vi "spectro.vi"() -> ()   [LabVIEW 2016]
uses:
  <vilib>/Analysis/baseanly.llb/Mean (DBL).vi
  <vilib>/Utility/file.llb/Write Delimited Spreadsheet (string).vi
  <vilib>/Utility/file.llb/Write Delimited Spreadsheet (DBL).vi
  <vilib>/Analysis/NI_AALBase.lvlib
panel:
  in  "stop":bool
  in  "Tab Control":enum32{"medir", "Mover"}(tab)
  out "Offset":dbl
  out "val act":dbl
  out "Valor y prom":dbl
  in  "num. med.":dbl
  out "XY Graph":cluster{dbl[], dbl[]}(graph)
  in  "iniciar":bool
  out "posicion":dbl
  in  "intervalo":dbl
  in  "Fin":dbl=100.0 min=100.0 max=15000.0
  in  "Inicio":dbl
  in  "offset":dbl=2000.0
  out "Longitud de onda actual":dbl
  in  "Mover":bool
  in  "Mover Monocromador":dbl
  in  "aceptar posición act.":bool
  in  "Posición actual":dbl
  # "Mover Monocromador"
  # "Definir Posición Actual"
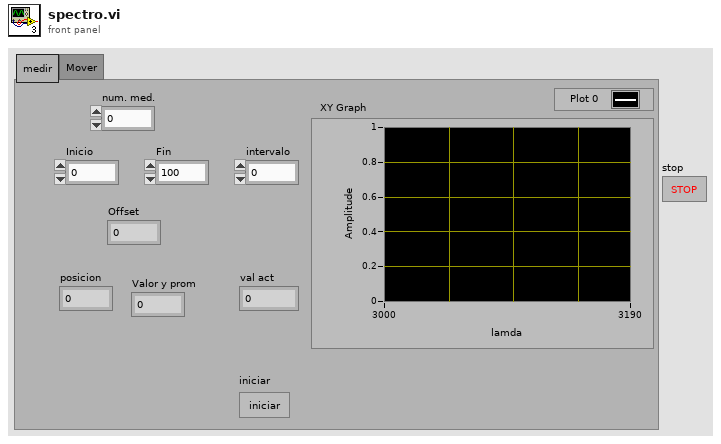
[diagram p1: front panel]
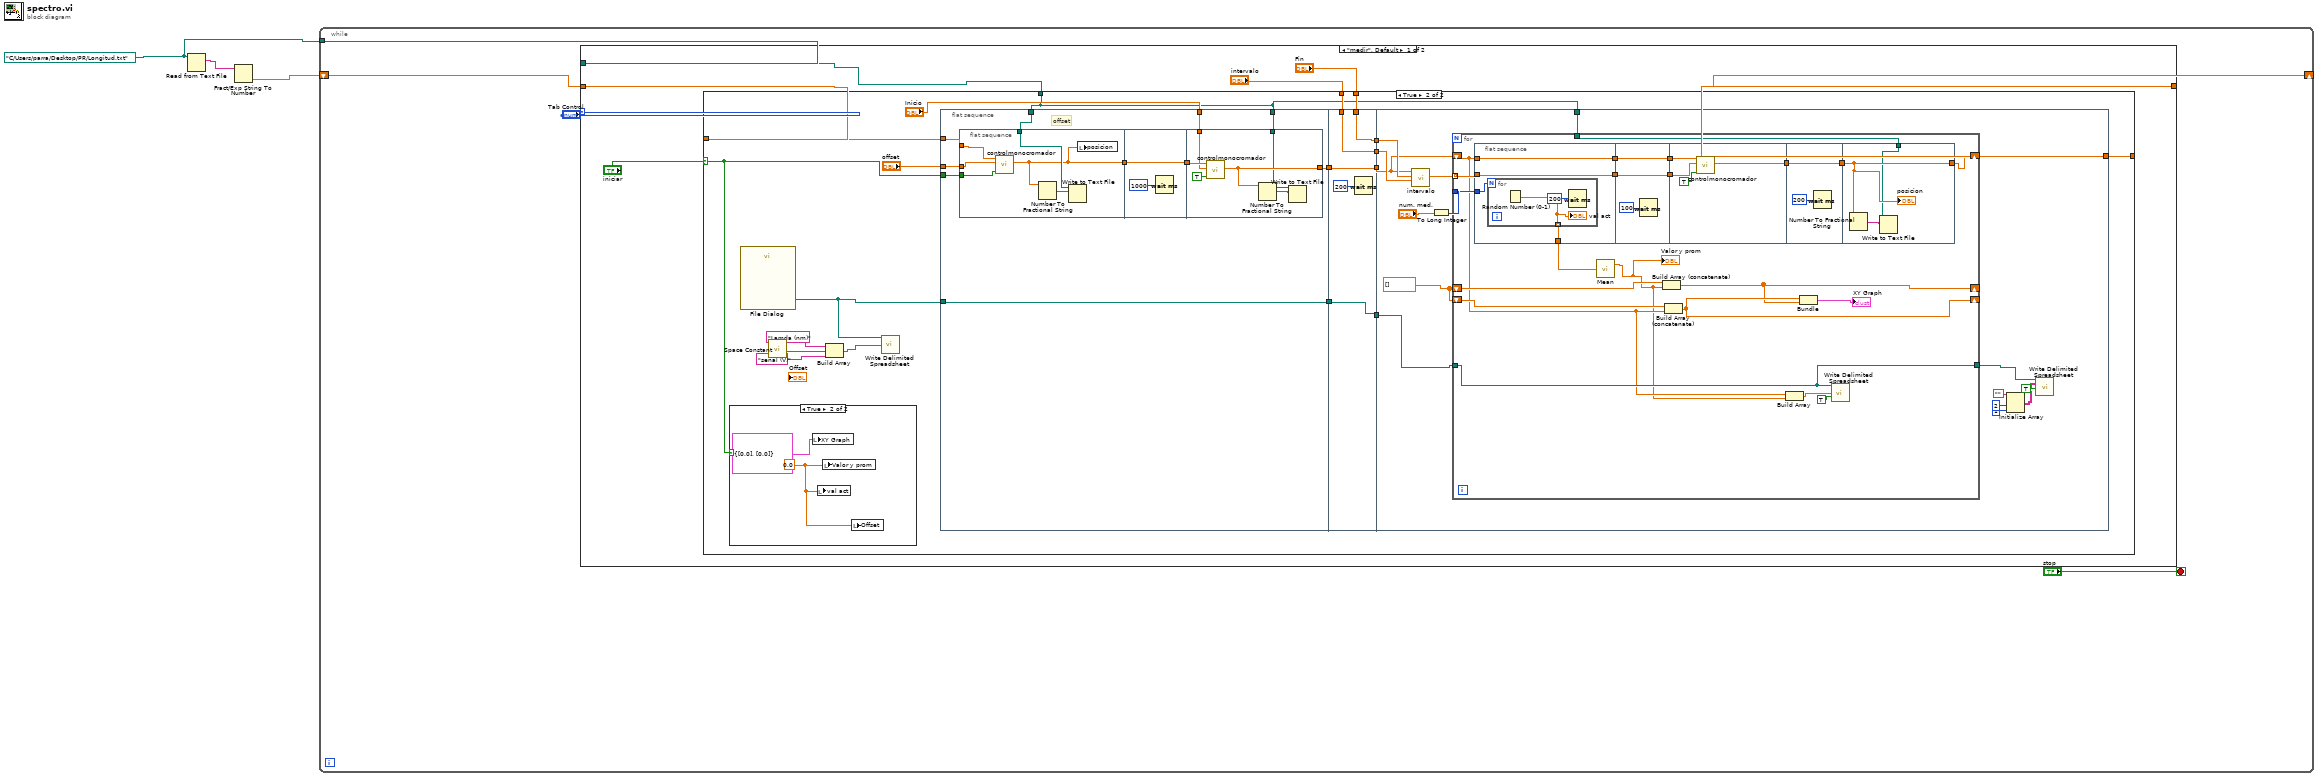
[diagram p0: block diagram]
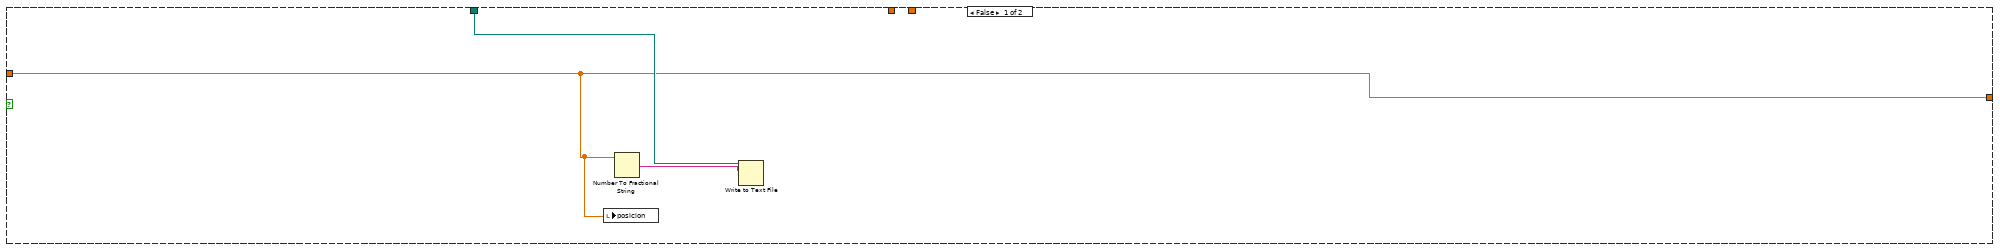
[diagram p2: hidden frame]
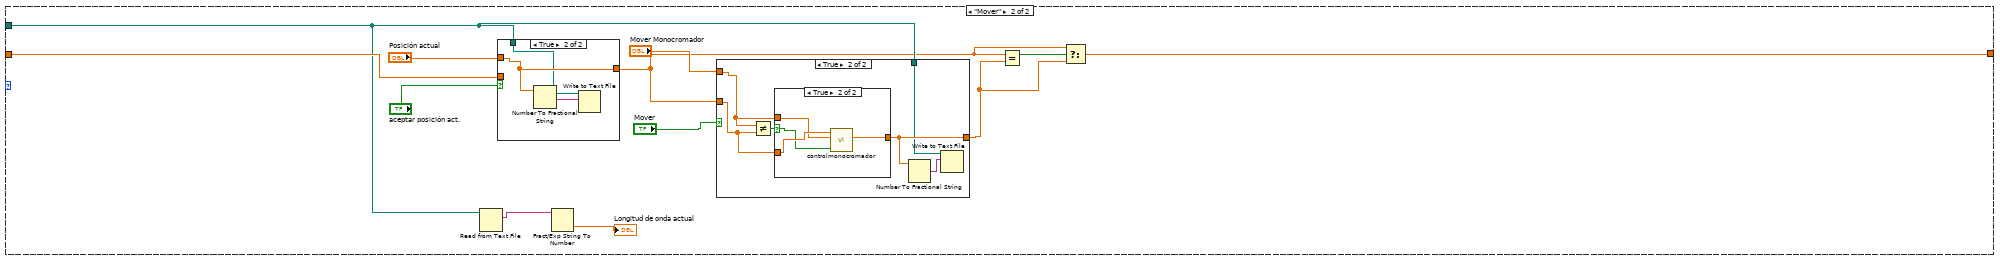
[diagram p4: hidden frame]
diagram:
  w1 = path "C:/Users/parra/Desktop/PR/Longitud.txt" ("file (use dialog)")
  n1 = Read from Text File(file (use dialog)=w1) -> (text=w3:string)  [unwired: 3 in, 3 out]
  n2 = Fract/Exp String To Number(string=w3) -> (number=w2:dbl)  [unwired: 3 in, 1 out]
  n3 = while {
    shift-right: [w4] -> _
    shift-left: w2 -> [w5]
    tunnel: w1 -> [w6]
    stop <- "stop" stop-if-true
    n4 = case shown="\"medir\", Default" "Tab Control" {
      tunnel: w6 -> [w13 w127]
      tunnel: w5 -> [w14 w132]
      tunnel: [w10 w123] -> w4
      frame "medir", Default {
        n5 = case shown="True" "iniciar" {
          selector: "iniciar" -> [_ w19]
          tunnel: w14 -> [w15 w35]
          tunnel: w13 -> [w17 w27]
          tunnel: "Fin" -> [_ w30]
          tunnel: "intervalo" -> [_ w28]
          tunnel: [w15 w26] -> w10
          frame False {
            n6 = local write "posicion"(w15) -> ()
            n7 = Number To Fractional String(number=w15) -> (F-format string=w16:string)  [unwired: 3 in]
            n8 = Write to Text File(file (use dialog)=w17, text=w16) -> ()  [unwired: 2 in, 3 out]
          }
          frame True {
            n9 = case shown="True" w19 {
              frame False {
              }
              frame True {
                w37 = 0.0 ("Valor y prom")
                n10 = local write "XY Graph"(cluster{dbl[], dbl[]} {[0.0], [0.0]} ("XY Graph")) -> ()
                n11 = local write "val act"(w37) -> ()
                n12 = local write "Valor y prom"(w37) -> ()
                n13 = local write "Offset"(w37) -> ()
              }
            }
            n14 = call "File Dialog"() -> ("selected path"=w23:path)  [unwired: 12 in, 3 out]
            n15 = call <vilib>:"Space Constant.vi"() -> ("String"=w21:string)
            n16 = Build Array("Lamda (nm)", w21, "señal (V)" ("element")) -> (w18:string[])
            n17 = call-poly <vilib>:"Write Delimited Spreadsheet.vi"("file path (dialog if empty)"=w23, "1D data"=w18) -> ()  [unwired: 12 in, 2 out]
            n18 = flat-sequence {
              tunnel: w35 -> [w48]
              tunnel: "offset" -> [w47]
              tunnel: w19 -> [w46]
              tunnel: w27 -> [w45]
              tunnel: "Inicio" -> [w42]
              tunnel: w27 -> [w41]
              tunnel: [w40] -> w33
              tunnel: w23 -> [w39]
              tunnel: [w39] -> w24
              tunnel: w33 -> [w67]
              tunnel: [w67] -> w32
              tunnel: [w65] -> w31
              tunnel: w30 -> [w65]
              tunnel: w28 -> [w64]
              tunnel: [w64] -> w29
              tunnel: [w63] -> w25
              tunnel: w24 -> [w63]
              tunnel: w32 -> [w80]
              tunnel: w31 -> [w83]
              tunnel: w29 -> [w82]
              tunnel: w27 -> [w79]
              tunnel: [w78] -> w26
              tunnel: w25 -> [w74]
              frame #0 {
                # "offset"
                n19 = flat-sequence {
                  tunnel: w48 -> [w54]
                  tunnel: w47 -> [w53]
                  tunnel: w46 -> [w49]
                  tunnel: w45 -> [w51]
                  tunnel: [w50] -> w44
                  tunnel: w44 -> [w56]
                  tunnel: [w56] -> w43
                  tunnel: w43 -> [w62]
                  tunnel: w42 -> [w61]
                  tunnel: [w59] -> w40
                  tunnel: w41 -> [w58]
                  frame #0 {
                    n20 = call "controlmonocromador.vi"(8:"inicio"=w49, "fin"=w53, 11:"inicio"=w54) -> ("Longitud actual"=w50:dbl)  [unwired: 8 in]
                    n21 = Number To Fractional String(number=w50) -> (F-format string=w52:string)  [unwired: 3 in]
                    n22 = Write to Text File(file (use dialog)=w51, text=w52) -> ()  [unwired: 2 in, 3 out]
                    n23 = local write "posicion"(w50) -> ()
                  }
                  frame #1 {
                    n24 = Wait (ms)(milliseconds to wait=u32 1000) -> ()  [unwired: 1 out]
                  }
                  frame #2 {
                    n25 = call "controlmonocromador.vi"(8:"inicio"=TRUE ("inicio"), "fin"=w61, 11:"inicio"=w62) -> ("Longitud actual"=w59:dbl)  [unwired: 8 in]
                    n26 = Number To Fractional String(number=w59) -> (F-format string=w60:string)  [unwired: 3 in]
                    n27 = Write to Text File(file (use dialog)=w58, text=w60) -> ()  [unwired: 2 in, 3 out]
                  }
                }
              }
              frame #1 {
                n28 = Wait (ms)(milliseconds to wait=u32 200) -> ()  [unwired: 1 out]
              }
              frame #2 {
                w75 = dbl[] []
                n29 = call "intervalo.vi"("Intervalo"=w82, "Final"=w83, "inicio"=w80) -> ("Array"=w81:dbl[])  [unwired: 8 in]
                n30 = To Long Integer(number="num. med.") -> (32bit integer=w76:i32)
                n31 = for {
                  tunnel: w81 -> [w104] mode=indexing
                  shift-right: [w91] -> w78
                  shift-left: w80 -> [w85]
                  tunnel: w79 -> [w101]
                  tunnel: w76 -> [w100]
                  shift-right: [w89] -> _
                  shift-left: w75 -> [w98]
                  shift-right: [w90] -> _
                  shift-left: w75 -> [w92]
                  tunnel: w74 -> [w88]
                  tunnel: [w88] -> w73
                  n32 = flat-sequence {
                    tunnel: w104 -> [w107]
                    tunnel: w85 -> [w108]
                    tunnel: [w108] -> w97
                    tunnel: [w107] -> w95
                    tunnel: w100 -> [w106]
                    tunnel: [w105] -> w99
                    tunnel: w97 -> [w113]
                    tunnel: [w113] -> w96
                    tunnel: w95 -> [w112]
                    tunnel: [w112] -> w94
                    tunnel: [w114] -> w103
                    tunnel: w96 -> [w117]
                    tunnel: w94 -> [w116]
                    tunnel: w103 -> [w119]
                    tunnel: [w119] -> w102
                    tunnel: [w121] -> w91
                    tunnel: w102 -> [w121]
                    tunnel: w101 -> [w120]
                    frame #0 {
                      n33 = for {
                        N: w106 -> [_]
                        tunnel: [w109] -> w105 mode=indexing
                        n34 = Random Number (0-1)() -> (number: 0 to 1=w109:dbl)
                        "val act" <- w109
                        n35 = Wait (ms)(milliseconds to wait=u32 200) -> ()  [unwired: 1 out]
                      }
                    }
                    frame #1 {
                      n36 = Wait (ms)(milliseconds to wait=u32 100) -> ()  [unwired: 1 out]
                    }
                    frame #2 {
                      n37 = call "controlmonocromador.vi"(8:"inicio"=TRUE ("inicio"), "fin"=w116, 11:"inicio"=w117) -> ("Longitud actual"=w114:dbl)  [unwired: 8 in]
                    }
                    frame #3 {
                      n38 = Wait (ms)(milliseconds to wait=u32 200) -> ()  [unwired: 1 out]
                    }
                    frame #4 {
                      n39 = Number To Fractional String(number=w121) -> (F-format string=w122:string)  [unwired: 3 in]
                      n40 = Write to Text File(file (use dialog)=w120, text=w122) -> ()  [unwired: 2 in, 3 out]
                      "posicion" <- w121
                    }
                  }
                  n41 = call-poly <vilib>:"Mean.vi"("X"=w99) -> ("mean"=w84:dbl)  [unwired: 1 out]
                  "Valor y prom" <- w84
                  n42 = Build Array (concatenate)(w98, w84) -> (w89:dbl[])
                  n43 = Build Array (concatenate)(w92, w85) -> (w90:dbl[])
                  n44 = Build Array(w85, w84) -> (w86:dbl[])
                  n45 = Bundle(w90, w89) -> (→"XY Graph":cluster{dbl[], dbl[]})  [unwired: 1 in]
                  n46 = call-poly <vilib>:"Write Delimited Spreadsheet.vi"("file path (dialog if empty)"=w88, "1D data"=w86, "append to file? (new file:F)"=TRUE) -> ()  [unwired: 11 in, 2 out]
                }
                n47 = Initialize Array("", 2 ("dimension size"), 1 ("dimension size")) -> (w68:string[][])
                n48 = call-poly <vilib>:"Write Delimited Spreadsheet.vi"("file path (dialog if empty)"=w73, "2D data"=w68, "append to file? (new file:F)"=TRUE) -> ()  [unwired: 11 in, 2 out]
              }
            }
          }
        }
      }
      frame "Mover" {
        n49 = Read from Text File(file (use dialog)=w127) -> (text=w131:string)  [unwired: 3 in, 3 out]
        n50 = case shown="True" "aceptar posición act." {
          tunnel: "Posición actual" -> [_ w149]
          tunnel: w127 -> [_ w148]
          tunnel: [w147 w149] -> w125
          tunnel: w132 -> [w147 _]
          frame False {
          }
          frame True {
            n51 = Number To Fractional String(number=w149) -> (F-format string=w150:string)  [unwired: 3 in]
            n52 = Write to Text File(file (use dialog)=w148, text=w150) -> ()  [unwired: 2 in, 3 out]
          }
        }
        n53 = Fract/Exp String To Number(string=w131) -> (number=→"Longitud de onda actual":dbl)  [unwired: 3 in, 1 out]
        n54 = case shown="True" "Mover" {
          tunnel: "Mover Monocromador" -> [_ w139]
          tunnel: w125 -> [w135 w140]
          tunnel: [w135 w138] -> w124
          tunnel: w127 -> [_ w136]
          frame False {
          }
          frame True {
            n55 = Not Equal?(x=w139, y=w140) -> (x != y?=w141:bool)
            n56 = case shown="True" w141 {
              selector: w141 -> [_ w144]
              tunnel: w140 -> [w142 w146]
              tunnel: w139 -> [_ w145]
              tunnel: [w142 w143] -> w138
              frame False {
              }
              frame True {
                n57 = call "controlmonocromador.vi"(8:"inicio"=w144, "fin"=w145, 11:"inicio"=w146) -> ("Longitud actual"=w143:dbl)  [unwired: 8 in]
              }
            }
            n58 = Number To Fractional String(number=w138) -> (F-format string=w137:string)  [unwired: 3 in]
            n59 = Write to Text File(file (use dialog)=w136, text=w137) -> ()  [unwired: 2 in, 3 out]
          }
        }
        n60 = Equal?(x=w125, y=w124) -> (x = y?=w126:bool)
        n61 = Select(t=w125, s=w126, f=w124) -> (s? t:f=w123:dbl)
      }
    }
  }
